vi "Untitled 7.vi"() -> ()   [LabVIEW 2026]
uses:
  <vilib>/Analysis/NI_AALBase.lvlib
  <vilib>/Analysis/1siggen.llb/Ramp Pattern by Samples.vi
  <vilib>/numeric/Random Number (Range) U64.vi
panel:
  out "Array 2":bool[](array[boolean])
  out "Array":bool[](array[boolean])
  in  "Lit":bool[](array[boolean])
  in  "Random Number":u8
  in  "Pressed":bool[](array[boolean])
  out "Waveform":waveform(dbl)(graph)
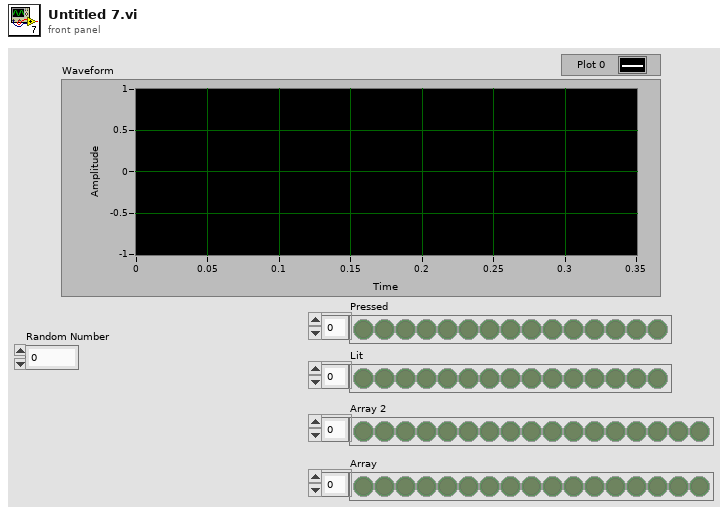
[diagram p1: front panel]
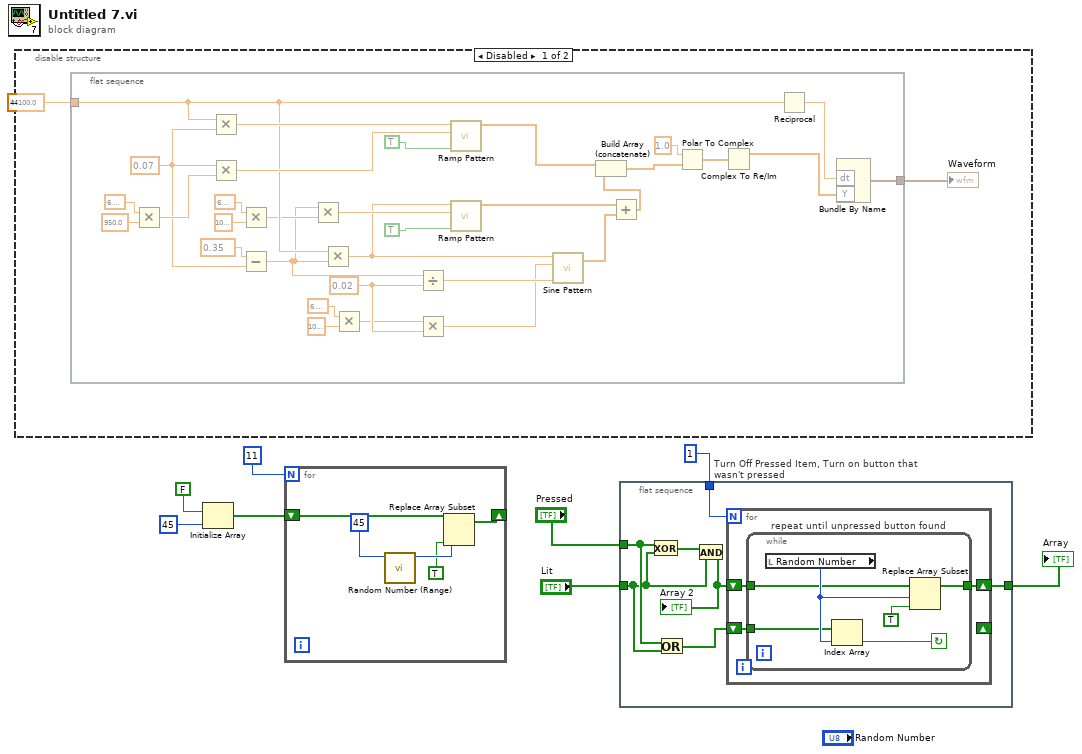
[diagram p0: block diagram]
diagram:
  n1 = disable-structure shown="Disabled" {
    frame Disabled {
      n2 = flat-sequence {
        tunnel: [w32] -> w9
        tunnel: 44100.0 ("rate") -> [w28]
        frame #0 {
          w16 = 0.02 ("y")
          w18 = 0.07 ("y")
          n3 = Multiply(x=6.283185307179586, y=950.0) -> (x*y=w39:dbl)
          n4 = Multiply(x=w28, y=w18) -> (x*y=w31:dbl)
          n5 = Multiply(x=w18, y=w39) -> (x*y=w37:dbl)
          n6 = Multiply(x=6.283185307179586, y=1000.0) -> (x*y=w24:dbl)
          n7 = Subtract(x=0.35 ("y"), y=w18) -> (x-y=w13:dbl)
          n8 = Multiply(x=w13, y=w24) -> (x*y=w30:dbl)
          n9 = Multiply(x=w28, y=w13) -> (x*y=w19:dbl)
          n10 = Multiply(x=6.283185307179586, y=1000.0) -> (x*y=w15:dbl)
          n11 = Divide(x=w13, y=w16) -> (x/y=w22:dbl)
          n12 = Multiply(x=w15, y=w16) -> (x*y=w14:dbl)
          n13 = call-poly <vilib>:"Ramp Pattern.vi"("exclude end?"=TRUE, "end"=w37, "samples"=w31) -> ("Ramp Pattern"=w40:dbl[])  [unwired: 7 in, 1 out]
          n14 = call-poly <vilib>:"Ramp Pattern.vi"("exclude end?"=TRUE, "end"=w30, "samples"=w19) -> ("Ramp Pattern"=w27:dbl[])  [unwired: 7 in, 1 out]
          n15 = call <vilib>:"Sine Pattern.vi"("cycles"=w22, "amplitude"=w14, "samples"=w19) -> ("Sinusoidal Pattern"=w17:dbl[])  [unwired: 1 in, 1 out]
          n16 = Add(x=w27, y=w17) -> (x+y=w11:dbl[])
          n17 = Build Array (concatenate)(w40, w11) -> (w12:dbl[])
          n18 = Polar To Complex(1:w12, 2:1.0 ("y")) -> (0:w35:cdb[])
          n19 = Complex To Re/Im(x + iy=w35) -> (x=w34:dbl[])  [unwired: 1 out]
          n20 = Reciprocal(x=w28) -> (1/x=w33:dbl)
          n21 = Bundle By Name("dt"=w33, "Y"=w34) -> (w32:waveform(dbl))  [unwired: 1 in]
        }
      }
      "Waveform" <- w9
    }
    frame Enabled {
    }
  }
  n22 = Initialize Array(FALSE, 45 ("dimension size")) -> (w6:bool[])
  n23 = for {
    N: 11 -> [_]
    shift-right: [w43] -> _
    shift-left: w6 -> [w44]
    n24 = call-poly <vilib>:"Random Number (Range).vi"("upper bound (100)"=u64 45) -> ("number"=w46:u64)  [unwired: 10 in]
    n25 = Replace Array Subset(array=w44, new element=TRUE, index=w46) -> (w43:bool[])
  }
  n26 = flat-sequence "Turn Off Pressed Item, Turn on button that wasn't pressed" {
    tunnel: "Pressed" -> [w50]
    tunnel: [w53] -> w1
    tunnel: "Lit" -> [w49]
    tunnel: u16 1 ("Count") -> [w52]
    frame #0 {
      n27 = Exclusive Or(1:w49, 2:w50) -> (0:w54:bool[])
      n28 = Or(x=w50, y=w49) -> (x .or. y?=w48:bool[])
      n29 = And(x=w54, y=w49) -> (x .and. y?=w51:bool[])
      "Array 2" <- w51
      n30 = for {
        N: w52 -> [_]
        shift-right: [w56] -> w53
        shift-left: w51 -> [w57]
        shift-right: _ -> [_]
        shift-left: w48 -> [w55]
        n31 = while "repeat until unpressed button found" {
          tunnel: w57 -> [w59]
          tunnel: [w62] -> w56
          tunnel: w55 -> [w58]
          stop <- w63 continue-if-true
          n32 = local read "Random Number"() -> (w61:u8)
          n33 = Index Array(array=w58, index=w61) -> (element=w63:bool)
          n34 = Replace Array Subset(array=w59, new element=TRUE ("new element/subarray"), index=w61) -> (w62:bool[])
        }
      }
    }
  }
  "Array" <- w1
